vi "Condition_Production_count_Day.vi"(0 "Select STATION":string(combo)="ST 1", 1 "connection reference":T1, 2 "Shift":string(combo)="ALL", 3 "stack_holder_ID":string(combo)="ALL", 4 "Found Date":string[](array[string]), 5 "year":string(combo)="ST 1", 6 "Form Date":timestamp format="%<%Y-%m-%d>T", 7 "error in (no error)":errorcluster, 8 "To Date":timestamp format="%<%Y-%m-%d>T") -> (12 "Duration count":string[][](array[string]), 13 "error out":errorcluster, 15 "connection reference 2":T1, 18 "BD Count":string[][](array[string]))   [LabVIEW 2017]
uses:
  <vilib>/addons/database/Connection.llb/Conn ObjectReference.ctl
  <vilib>/addons/database/NI_Database_API.lvlib
panel:
  out "Table":string[][](array[string])
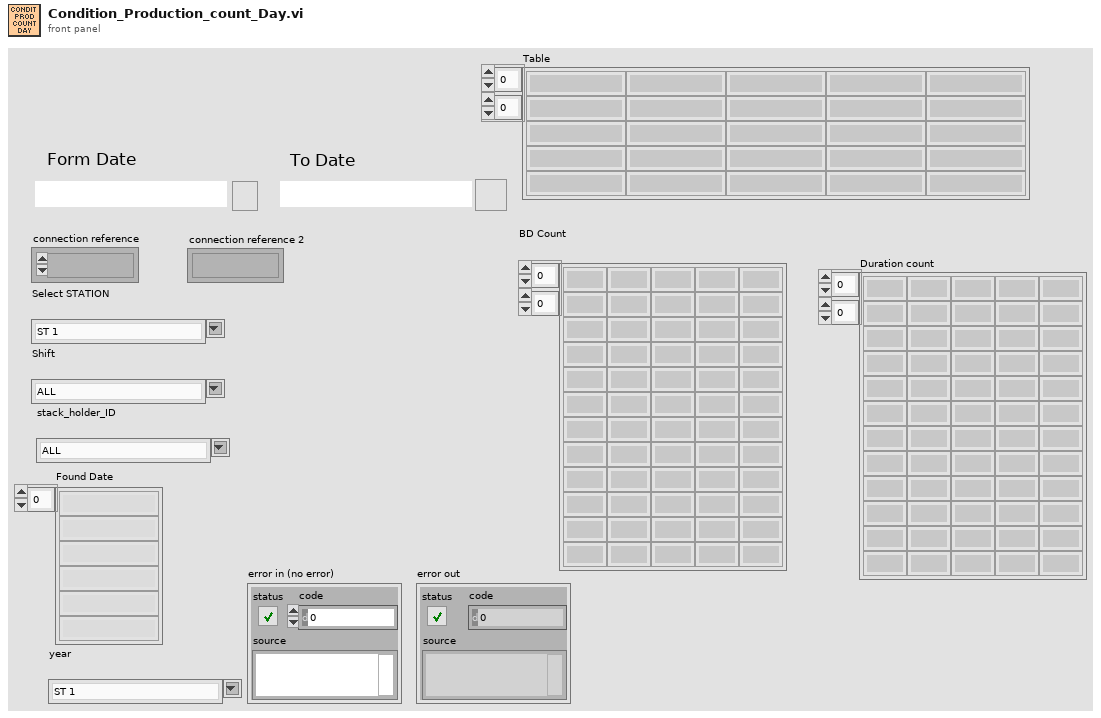
[diagram p1: front panel]
types:
  T1 = typedef "NI_Database_API.lvlib/Conn ObjectReference.ctl" = refnum<k1>
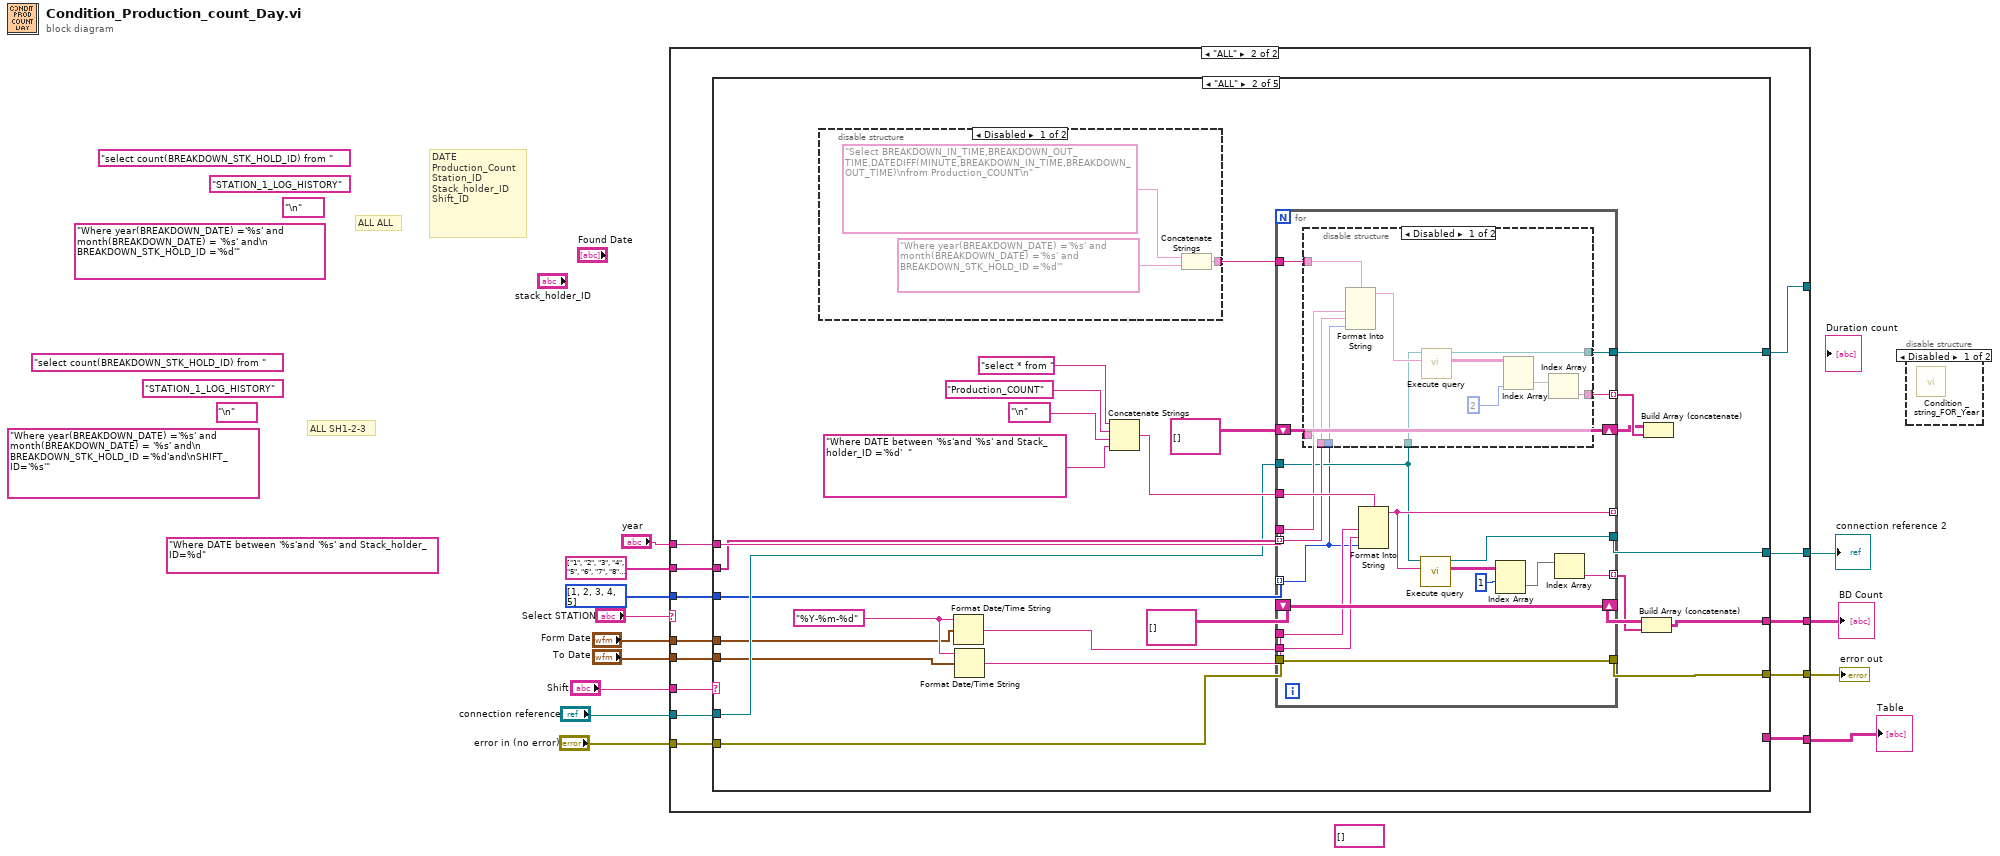
[diagram p0: block diagram]
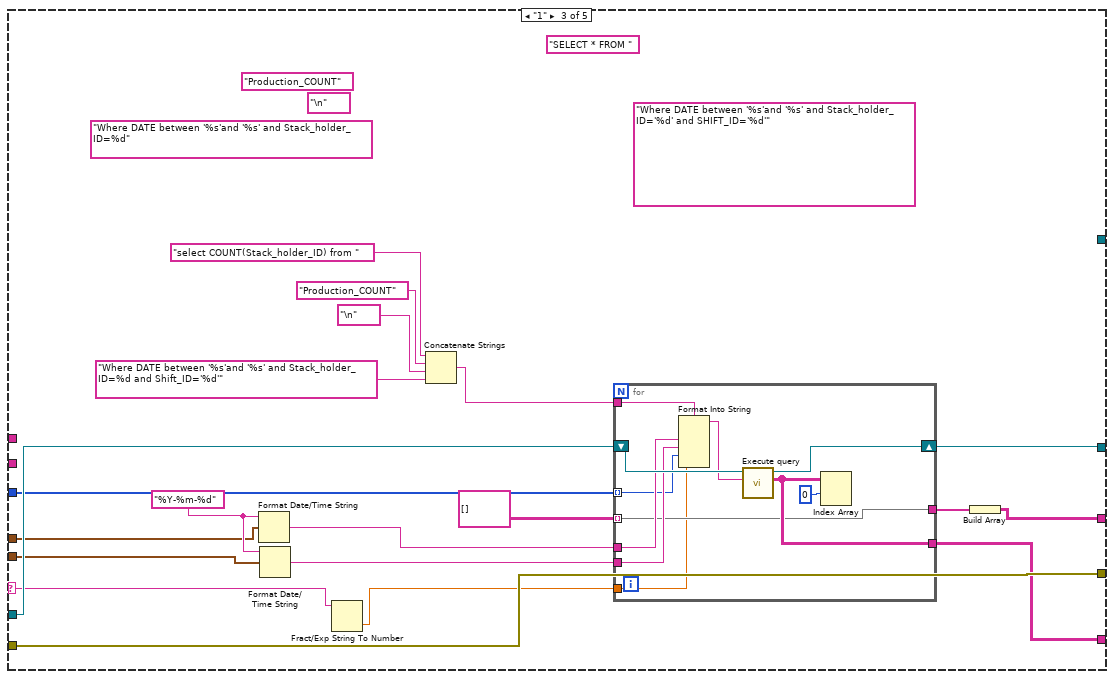
[diagram p7: hidden frame]
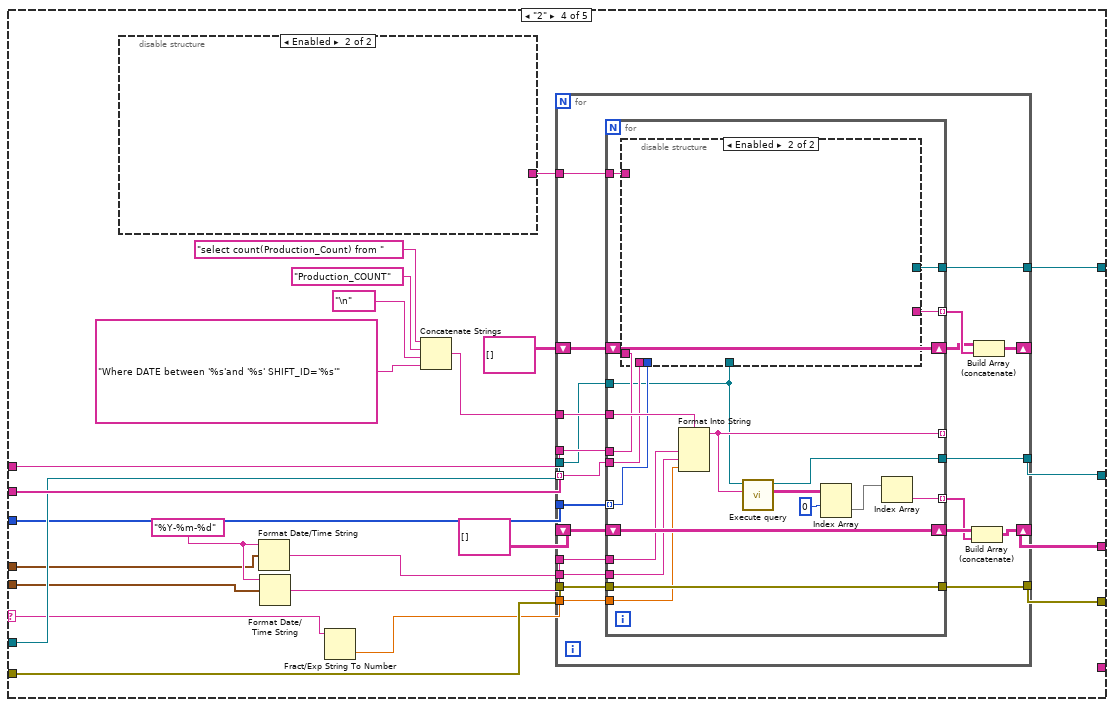
[diagram p8: hidden frame]
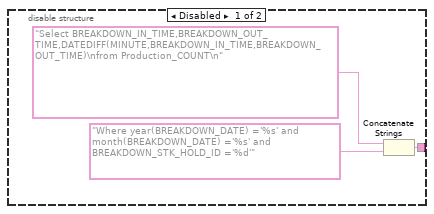
[diagram p9: hidden frame]
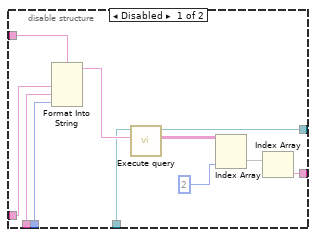
[diagram p10: hidden frame]
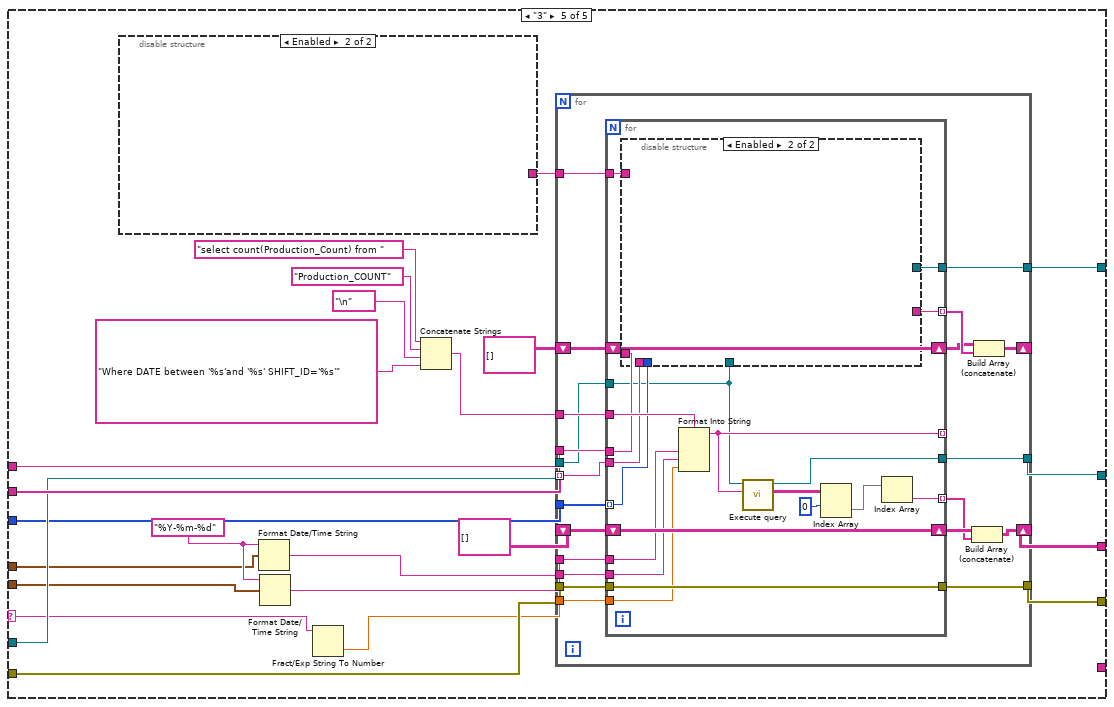
[diagram p11: hidden frame]
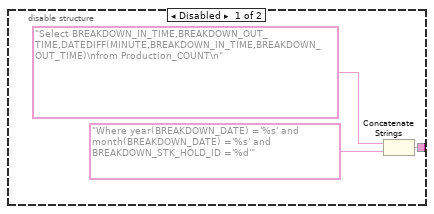
[diagram p12: hidden frame]
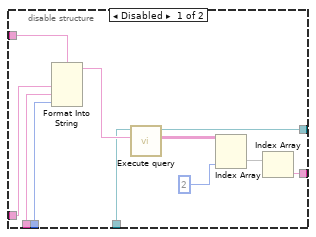
[diagram p13: hidden frame]
diagram:
  (unwired) "Where DATE between '%s'and '%s' and Stack_holder_ID=%d" ("condition")
  (unwired) "STATION_1_LOG_HISTORY" ("table")
  (unwired) "\n" ("string")
  (unwired) "select count(BREAKDOWN_STK_HOLD_ID) from " ("string")
  (unwired) "Where year(BREAKDOWN_DATE) ='%s' and month(BREAKDOWN_DATE) = '%s' and\n BREAKDOWN_STK_HOLD_ID ='%d'and\nSHIFT_ID='%s'" ("condition")
  (unwired) "STATION_1_LOG_HISTORY" ("table")
  (unwired) "\n" ("string")
  (unwired) "select count(BREAKDOWN_STK_HOLD_ID) from " ("string")
  (unwired) "Where year(BREAKDOWN_DATE) ='%s' and month(BREAKDOWN_DATE) = '%s' and\n BREAKDOWN_STK_HOLD_ID ='%d'" ("condition")
  (unwired) string[] [] ("Output Array")
  # "ALL SH1-2-3"
  # "ALL ALL"
  # "DATE\nProduction_Count\nStation_ID\nStack_holder_ID\nShift_ID"
  n1 = case shown="\"ALL\"" "Select STATION" {
    tunnel: "Shift" -> [_ w26]
    tunnel: "year" -> [_ w25]
    tunnel: string[] ["1", "2", "3", "4", "5", "6", "7", "8", "9", "10", "11", "12"] -> [_ w24]
    tunnel: [_ w23] -> w9
    tunnel: "connection reference" -> [_ w22]
    tunnel: [_ w21] -> w7
    tunnel: i32[] [1, 2, 3, 4, 5] -> [_ w20]
    tunnel: [_ w19] -> _
    tunnel: "error in (no error)" -> [_ w18]
    tunnel: [_ w17] -> w4
    tunnel: "Form Date" -> [_ w16]
    tunnel: "To Date" -> [_ w15]
    tunnel: [_ w14] -> w1
    frame "False", Default {
    }
    frame "ALL" {
      n2 = case shown="\"ALL\"" w26 {
        selector: w26 -> [_ _ w96 w120 w199]
        tunnel: w25 -> [_ w51 _ w137 w216]
        tunnel: w24 -> [_ w48 _ w134 w213]
        tunnel: [_ w52 w93 w138 w217] -> w23
        tunnel: w22 -> [w28 w47 w104 w133 w212]
        tunnel: [w28 w46 w103 w132 w211] -> w21
        tunnel: w20 -> [_ w45 w94 w131 w210]
        tunnel: [_ w42 _ w128 w207] -> w19
        tunnel: w18 -> [w27 w41 w102 w127 w206]
        tunnel: [w27 w40 w102 w126 w205] -> w17
        tunnel: w16 -> [_ w38 w100 w124 w203]
        tunnel: w15 -> [_ w37 w99 w123 w202]
        tunnel: [_ _ w88 _ _] -> w14
        frame "False", Default {
        }
        frame "ALL" {
          w39 = "%Y-%m-%d" ("time format string (%c)")
          n3 = disable-structure shown="Disabled" {
            disable-tunnel: [w86 _] -> w44
            frame Disabled {
              n4 = Concatenate Strings("Select BREAKDOWN_IN_TIME,BREAKDOWN_OUT_TIME,DATEDIFF(MINUTE,BREAKDOWN_IN_TIME,BREAKDOWN_OUT_TIME)\nfrom Production_COUNT\n" ("string"), "Where year(BREAKDOWN_DATE) ='%s' and month(BREAKDOWN_DATE) ='%s' and BREAKDOWN_STK_HOLD_ID ='%d'" ("condition")) -> (w86:string)
            }
            frame Enabled {
            }
          }
          n5 = Format Date/Time String(time format string (%c)=w39, seconds (now)=w38) -> (date/time string=w36:string)  [unwired: 1 in]
          n6 = Format Date/Time String(time format string (%c)=w39, seconds (now)=w37) -> (date/time string=w35:string)  [unwired: 1 in]
          n7 = Concatenate Strings("select * from " ("string"), "Production_COUNT" ("table"), "\n" ("string"), "Where DATE between '%s'and '%s' and Stack_holder_ID ='%d'  ") -> (w50:string)
          n8 = for {
            tunnel: w50 -> [w73]
            tunnel: w51 -> [w64]
            tunnel: w48 -> [w63] mode=indexing
            tunnel: [w72] -> _ mode=indexing
            tunnel: w47 -> [w62]
            tunnel: [w70] -> w46
            tunnel: w45 -> [w55] mode=indexing
            shift-right: [w71] -> w34
            shift-left: string[][] [] ("Output Array") -> [w71]
            tunnel: [w66] -> w33 mode=indexing
            tunnel: w44 -> [w65]
            tunnel: [w61] -> w42
            tunnel: [w60] -> w32 mode=indexing
            shift-right: [w59] -> w31
            shift-left: string[][] [] ("Output Array") -> [w59]
            tunnel: [w58] -> w40
            tunnel: w41 -> [w58]
            tunnel: w36 -> [w57]
            tunnel: w35 -> [w56]
            n9 = disable-structure shown="Disabled" {
              disable-tunnel: w65 -> [w83 _]
              disable-tunnel: w64 -> [w82 _]
              disable-tunnel: w63 -> [w81 _]
              disable-tunnel: w55 -> [w80 _]
              disable-tunnel: w62 -> [w79 _]
              disable-tunnel: [w76 _] -> w61
              disable-tunnel: [w75 _] -> w60
              frame Disabled {
                n10 = Format Into String(format string=w83, w82, w81, w80) -> (resulting string=w84:string)  [unwired: 2 in, 1 out]
                n11 = call "Execute query.vi"("String"=w84, "connection reference"=w79) -> ("Table"=w78:string[][], "connection reference 2"=w76:T1)  [unwired: 6 in, 2 out]
                n12 = Index Array(array=w78, index (col)=2 ("disabled index (col)")) -> (element=w77:string[])  [unwired: 1 in]
                n13 = Index Array(array=w77) -> (element=w75:string)  [unwired: 1 in]
              }
              frame Enabled {
              }
            }
            n14 = Format Into String(format string=w73, w57, w56, w55) -> (resulting string=w72:string)  [unwired: 2 in, 1 out]
            n15 = call "Execute query.vi"("String"=w72, "connection reference"=w62) -> ("Table"=w69:string[][], "connection reference 2"=w70:T1)  [unwired: 6 in, 2 out]
            n16 = Index Array(array=w69, index (row)=1 ("disabled index (col)")) -> (element=w67:string[])  [unwired: 1 in]
            n17 = Index Array(array=w67) -> (element=w66:string)  [unwired: 1 in]
          }
          n18 = Build Array (concatenate)(w34, w33) -> (w52:string[][])
          n19 = Build Array (concatenate)(w31, w32) -> ()  [unwired: 1 out]
        }
        frame "1" {
          (unwired) "Where DATE between '%s'and '%s' and Stack_holder_ID='%d' and SHIFT_ID='%d'" ("condition")
          (unwired) "Production_COUNT" ("table")
          (unwired) "\n" ("string")
          (unwired) "Where DATE between '%s'and '%s' and Stack_holder_ID=%d" ("condition")
          w101 = "%Y-%m-%d" ("time format string (%c)")
          (unwired) "SELECT * FROM " ("string")
          n20 = Format Date/Time String(time format string (%c)=w101, seconds (now)=w100) -> (date/time string=w98:string)  [unwired: 1 in]
          n21 = Format Date/Time String(time format string (%c)=w101, seconds (now)=w99) -> (date/time string=w97:string)  [unwired: 1 in]
          n22 = Fract/Exp String To Number(string=w96) -> (number=w95:dbl)  [unwired: 3 in, 1 out]
          n23 = Concatenate Strings("select COUNT(Stack_holder_ID) from " ("string"), "Production_COUNT" ("table"), "\n" ("string"), "Where DATE between '%s'and '%s' and Stack_holder_ID=%d and Shift_ID='%d'" ("condition")) -> (w105:string)
          n24 = for {
            tunnel: w105 -> [w118]
            tunnel: w98 -> [w115]
            tunnel: w97 -> [w114]
            tunnel: w95 -> [w108]
            tunnel: [w111] -> w88
            shift-right: [w116] -> w103
            shift-left: w104 -> [w117]
            tunnel: w94 -> [w109] mode=indexing
            tunnel: [w110] -> w92
            tunnel: string[][] [] ("Output Array") -> [w110] mode=indexing
            n25 = Format Into String(format string=w118, w115, w114, w109, w108) -> (resulting string=w113:string)  [unwired: 2 in, 1 out]
            n26 = call "Execute query.vi"("String"=w113, "connection reference"=w117) -> ("Table"=w111:string[][], "connection reference 2"=w116:T1)  [unwired: 6 in, 2 out]
            n27 = Index Array(array=w111, index (row)=0 ("disabled index (col)")) -> ()  [unwired: 1 in, 1 out]
          }
          n28 = Build Array(w92) -> (w93:string[][])
        }
        frame "2" {
          w125 = "%Y-%m-%d" ("time format string (%c)")
          n29 = disable-structure shown="Enabled" {
            disable-tunnel: [w144 _] -> w130
            frame Disabled {
              n30 = Concatenate Strings("Select BREAKDOWN_IN_TIME,BREAKDOWN_OUT_TIME,DATEDIFF(MINUTE,BREAKDOWN_IN_TIME,BREAKDOWN_OUT_TIME)\nfrom Production_COUNT\n" ("string"), "Where year(BREAKDOWN_DATE) ='%s' and month(BREAKDOWN_DATE) ='%s' and BREAKDOWN_STK_HOLD_ID ='%d'" ("condition")) -> (w144:string)
            }
            frame Enabled {
            }
          }
          n31 = Format Date/Time String(time format string (%c)=w125, seconds (now)=w124) -> (date/time string=w122:string)  [unwired: 1 in]
          n32 = Format Date/Time String(time format string (%c)=w125, seconds (now)=w123) -> (date/time string=w121:string)  [unwired: 1 in]
          n33 = Fract/Exp String To Number(string=w120) -> (number=w119:dbl)  [unwired: 3 in, 1 out]
          n34 = Concatenate Strings("select count(Production_Count) from " ("string"), "Production_COUNT" ("table"), "\n" ("string"), "Where DATE between '%s'and '%s' SHIFT_ID='%s'" ("condition")) -> (w136:string)
          n35 = for {
            tunnel: w137 -> [w166]
            tunnel: w136 -> [w165]
            tunnel: w134 -> [w163] mode=indexing
            tunnel: w133 -> [w162]
            tunnel: [w161] -> w132
            tunnel: w131 -> [w160]
            shift-right: [w158] -> w138
            shift-left: string[][] [] ("Output Array") -> [w164]
            tunnel: w130 -> [w156]
            tunnel: [w155] -> w128
            shift-right: [w151] -> _
            shift-left: string[][] [] ("Output Array") -> [w152]
            tunnel: [w150] -> w126
            tunnel: w127 -> [w149]
            tunnel: w122 -> [w148]
            tunnel: w121 -> [w147]
            tunnel: w119 -> [w146]
            n36 = for {
              tunnel: w165 -> [w186]
              tunnel: w166 -> [w177]
              tunnel: w163 -> [w176]
              tunnel: [w185] -> _ mode=indexing
              tunnel: w162 -> [w174]
              tunnel: [w183] -> w161
              tunnel: w160 -> [w175] mode=indexing
              shift-right: [w184] -> w159
              shift-left: w164 -> [w184]
              tunnel: [w179] -> w157 mode=indexing
              tunnel: w156 -> [w178]
              tunnel: [w173] -> w155
              tunnel: [w172] -> w154 mode=indexing
              shift-right: [w171] -> w153
              shift-left: w152 -> [w171]
              tunnel: [w170] -> w150
              tunnel: w149 -> [w170]
              tunnel: w148 -> [w169]
              tunnel: w147 -> [w168]
              tunnel: w146 -> [w167]
              n37 = disable-structure shown="Enabled" {
                disable-tunnel: w178 -> [w196 _]
                disable-tunnel: w177 -> [w195 _]
                disable-tunnel: w176 -> [w194 _]
                disable-tunnel: w175 -> [w193 _]
                disable-tunnel: w174 -> [w192 _]
                disable-tunnel: [w189 _] -> w173
                disable-tunnel: [w188 _] -> w172
                frame Disabled {
                  n38 = Format Into String(format string=w196, w195, w194, w193) -> (resulting string=w197:string)  [unwired: 2 in, 1 out]
                  n39 = call "Execute query.vi"("String"=w197, "connection reference"=w192) -> ("Table"=w191:string[][], "connection reference 2"=w189:T1)  [unwired: 6 in, 2 out]
                  n40 = Index Array(array=w191, index (col)=2 ("disabled index (col)")) -> (element=w190:string[])  [unwired: 1 in]
                  n41 = Index Array(array=w190) -> (element=w188:string)  [unwired: 1 in]
                }
                frame Enabled {
                }
              }
              n42 = Format Into String(format string=w186, w169, w168, w167) -> (resulting string=w185:string)  [unwired: 2 in, 1 out]
              n43 = call "Execute query.vi"("String"=w185, "connection reference"=w174) -> ("Table"=w182:string[][], "connection reference 2"=w183:T1)  [unwired: 6 in, 2 out]
              n44 = Index Array(array=w182, index (row)=0 ("disabled index (col)")) -> (element=w180:string[])  [unwired: 1 in]
              n45 = Index Array(array=w180) -> (element=w179:string)  [unwired: 1 in]
            }
            n46 = Build Array (concatenate)(w159, w157) -> (w158:string[][])
            n47 = Build Array (concatenate)(w153, w154) -> (w151:string[][])
          }
        }
        frame "3" {
          w204 = "%Y-%m-%d" ("time format string (%c)")
          n48 = disable-structure shown="Enabled" {
            disable-tunnel: [w223 _] -> w209
            frame Disabled {
              n49 = Concatenate Strings("Select BREAKDOWN_IN_TIME,BREAKDOWN_OUT_TIME,DATEDIFF(MINUTE,BREAKDOWN_IN_TIME,BREAKDOWN_OUT_TIME)\nfrom Production_COUNT\n" ("string"), "Where year(BREAKDOWN_DATE) ='%s' and month(BREAKDOWN_DATE) ='%s' and BREAKDOWN_STK_HOLD_ID ='%d'" ("condition")) -> (w223:string)
            }
            frame Enabled {
            }
          }
          n50 = Format Date/Time String(time format string (%c)=w204, seconds (now)=w203) -> (date/time string=w201:string)  [unwired: 1 in]
          n51 = Format Date/Time String(time format string (%c)=w204, seconds (now)=w202) -> (date/time string=w200:string)  [unwired: 1 in]
          n52 = Fract/Exp String To Number(string=w199) -> (number=w198:dbl)  [unwired: 3 in, 1 out]
          n53 = Concatenate Strings("select count(Production_Count) from " ("string"), "Production_COUNT" ("table"), "\n" ("string"), "Where DATE between '%s'and '%s' SHIFT_ID='%s'" ("condition")) -> (w215:string)
          n54 = for {
            tunnel: w216 -> [w245]
            tunnel: w215 -> [w244]
            tunnel: w213 -> [w242] mode=indexing
            tunnel: w212 -> [w241]
            tunnel: [w240] -> w211
            tunnel: w210 -> [w239]
            shift-right: [w237] -> w217
            shift-left: string[][] [] ("Output Array") -> [w243]
            tunnel: w209 -> [w235]
            tunnel: [w234] -> w207
            shift-right: [w230] -> _
            shift-left: string[][] [] ("Output Array") -> [w231]
            tunnel: [w229] -> w205
            tunnel: w206 -> [w228]
            tunnel: w201 -> [w227]
            tunnel: w200 -> [w226]
            tunnel: w198 -> [w225]
            n55 = for {
              tunnel: w244 -> [w265]
              tunnel: w245 -> [w256]
              tunnel: w242 -> [w255]
              tunnel: [w264] -> _ mode=indexing
              tunnel: w241 -> [w253]
              tunnel: [w262] -> w240
              tunnel: w239 -> [w254] mode=indexing
              shift-right: [w263] -> w238
              shift-left: w243 -> [w263]
              tunnel: [w258] -> w236 mode=indexing
              tunnel: w235 -> [w257]
              tunnel: [w252] -> w234
              tunnel: [w251] -> w233 mode=indexing
              shift-right: [w250] -> w232
              shift-left: w231 -> [w250]
              tunnel: [w249] -> w229
              tunnel: w228 -> [w249]
              tunnel: w227 -> [w248]
              tunnel: w226 -> [w247]
              tunnel: w225 -> [w246]
              n56 = disable-structure shown="Enabled" {
                disable-tunnel: w257 -> [w275 _]
                disable-tunnel: w256 -> [w274 _]
                disable-tunnel: w255 -> [w273 _]
                disable-tunnel: w254 -> [w272 _]
                disable-tunnel: w253 -> [w271 _]
                disable-tunnel: [w268 _] -> w252
                disable-tunnel: [w267 _] -> w251
                frame Disabled {
                  n57 = Format Into String(format string=w275, w274, w273, w272) -> (resulting string=w276:string)  [unwired: 2 in, 1 out]
                  n58 = call "Execute query.vi"("String"=w276, "connection reference"=w271) -> ("Table"=w270:string[][], "connection reference 2"=w268:T1)  [unwired: 6 in, 2 out]
                  n59 = Index Array(array=w270, index (col)=2 ("disabled index (col)")) -> (element=w269:string[])  [unwired: 1 in]
                  n60 = Index Array(array=w269) -> (element=w267:string)  [unwired: 1 in]
                }
                frame Enabled {
                }
              }
              n61 = Format Into String(format string=w265, w248, w247, w246) -> (resulting string=w264:string)  [unwired: 2 in, 1 out]
              n62 = call "Execute query.vi"("String"=w264, "connection reference"=w253) -> ("Table"=w261:string[][], "connection reference 2"=w262:T1)  [unwired: 6 in, 2 out]
              n63 = Index Array(array=w261, index (row)=0 ("disabled index (col)")) -> (element=w259:string[])  [unwired: 1 in]
              n64 = Index Array(array=w259) -> (element=w258:string)  [unwired: 1 in]
            }
            n65 = Build Array (concatenate)(w238, w236) -> (w237:string[][])
            n66 = Build Array (concatenate)(w232, w233) -> (w230:string[][])
          }
        }
      }
    }
  }
  "BD Count" <- w9
  "connection reference 2" <- w7
  "error out" <- w4
  "Table" <- w1
  n67 = disable-structure shown="Disabled" {
    frame Disabled {
      n68 = call "Condition _string_FOR_Year.vi"() -> ()  [unwired: 16 in, 4 out]
    }
    frame Enabled {
    }
  }
